vi "Init Task.vi"(6 "line grouping":i32(ring) items=["one channel for each line", "one channel for all lines"], 7 "counter":tag, 8 "error in (no error)":errorcluster, 9 "name":string, 10 "physical channels":tag, 11 "DAQmxTaskAICurrent in":refnum<class "DAQmxTaskAICurrent.lvclass">) -> (0 "error out":errorcluster, 3 "DAQmxTaskAICurrent out":refnum<class "DAQmxTaskAICurrent.lvclass">)   [LabVIEW 2015, in "DAQmxTaskAICurrent.lvclass"]
uses:
  DAQmxTaskAICurrent.lvclass
  DAQmxTask.lvclass/DAQmxTask.ctl
  <vilib>/DAQmx/create/channels.llb/DAQmx Create Channel (AI-Current-Basic).vi
  DAQmxTask.lvclass
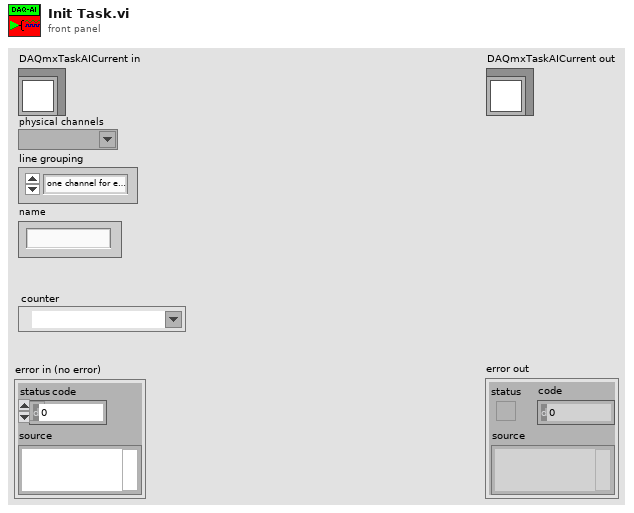
[diagram p1: front panel]
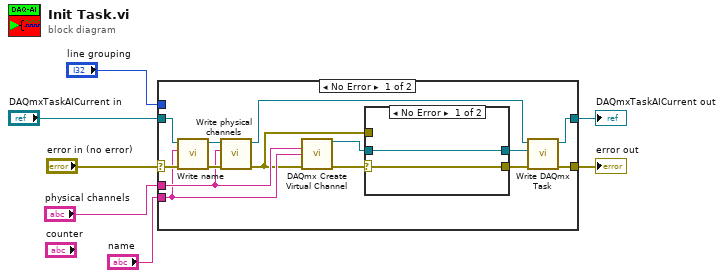
[diagram p0: block diagram]
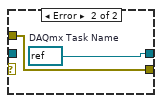
[diagram p2: hidden frame]
diagram:
  n1 = case shown="No Error" "error in (no error)" {
    selector: "error in (no error)" -> [w21 w27]
    tunnel: [w13 w27] -> w6
    tunnel: [w14 w26] -> w5
    tunnel: "name" -> [w16 _]
    tunnel: "physical channels" -> [w17 _]
    tunnel: "line grouping" -> [_ _]
    tunnel: "DAQmxTaskAICurrent in" -> [w15 w26]
    frame No Error {
      n2 = call "Write name.vi"("error in (no error)"=w21, "name"=w16, "DAQmxTask in"=w15) -> ("error out"=w19:errorcluster, "DAQmxTask out"=w20:refnum<class "DAQmxTaskAICurrent.lvclass">)  [unwired: 7 in]
      n3 = call "Write physical channels.vi"("error in (no error)"=w19, "physical channels"=w17, "DAQmxTask in"=w20) -> ("error out"=w10:errorcluster, "DAQmxTask out"=w18:refnum<class "DAQmxTaskAICurrent.lvclass">)  [unwired: 7 in]
      n4 = call-poly <vilib>:"DAQmx Create Virtual Channel.vi"("physical channels"=w17, "name to assign"=w16, "error in"=w10) -> ("task out"=w12:refnum<k21>, "error out"=w11:errorcluster)  [unwired: 11 in]
      n5 = case shown="No Error" w11 {
        selector: w11 -> [w22 _]
        tunnel: [w23 w24] -> w9
        tunnel: w12 -> [w23 _]
        tunnel: [w22 w25] -> w8
        tunnel: w10 -> [_ w25]
        frame No Error {
        }
        frame Error {
          w24 = refnum<k21> refnum  # DAQmx Task Name
        }
      }
      n6 = call "Write DAQmx Task.vi"("error in (no error)"=w8, "DAQmx Task Name"=w9, "DAQmxTask in"=w18) -> ("error out"=w13:errorcluster, "DAQmxTask out"=w14:refnum<class "DAQmxTaskAICurrent.lvclass">)  [unwired: 7 in]
    }
    frame Error {
    }
  }
  "error out" <- w6
  "DAQmxTaskAICurrent out" <- w5
